vi "LVBlynk.vi"() -> ()   [LabVIEW 2014]
uses:
  utilities/BlynkLogs.vi
panel:
  in  "LED":bool
  out "Array":string[](array[string])
  in  "Notify":bool
  out "Log":string
  in  "Stop Button":bool
  out "Connected":bool
  in  "Auth Token from Blynk app":string="c3404b1e978b40fcbb409a59fc5da34b"
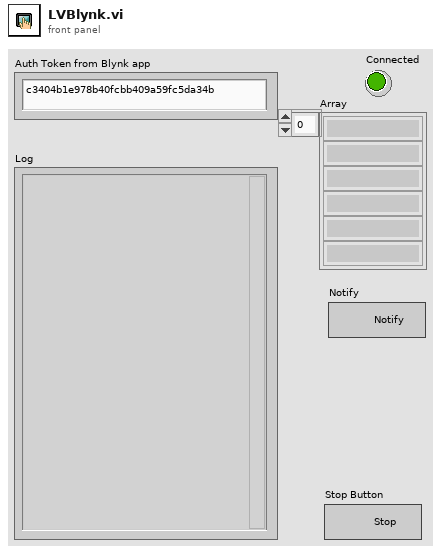
[diagram p1: front panel]
types:
  T1 = typedef "MsgType.ctl" = enum8{"RSP", "REGISTER", "LOGIN", "SAVE_PROF", "LOAD_PROF", "GET_TOKEN", "PING", "ACTIVATE", "DEACTIVATE", "REFRESH", "UNDEFINED0", "UNDEFINED1", "TWEET", "EMAIL", "NOTIFY", "BRIDGE", "UNDEFINED2", "UNDEFINED3", "UNDEFINED4", "UNDEFINED5", "HW"}
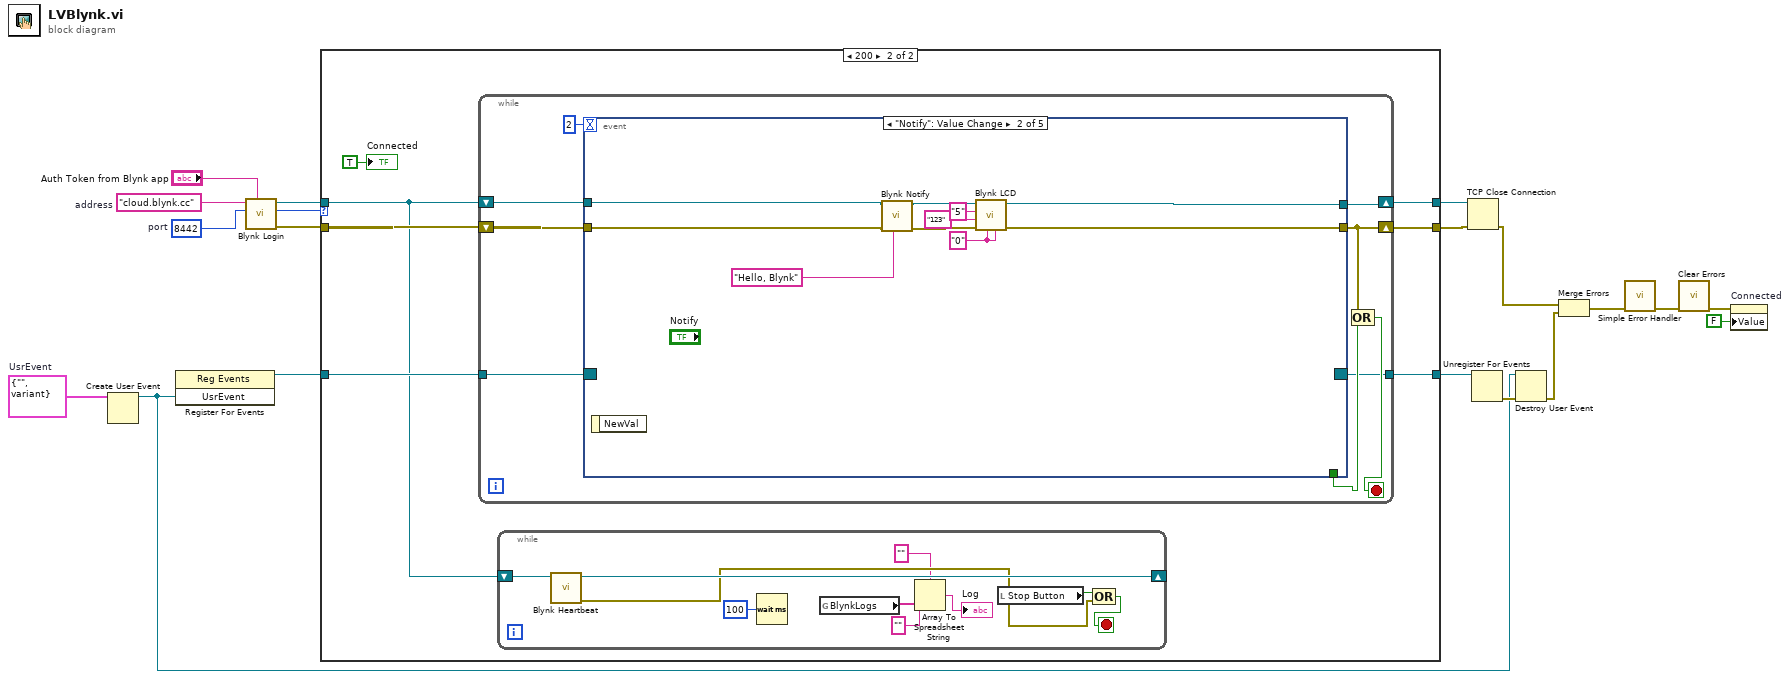
[diagram p0: block diagram]
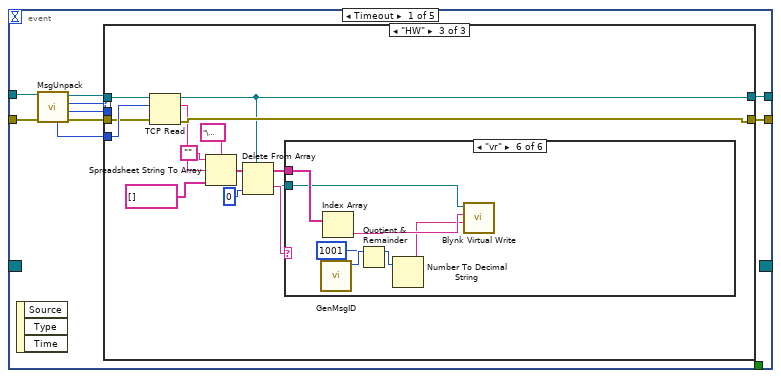
[diagram p3: hidden frame]
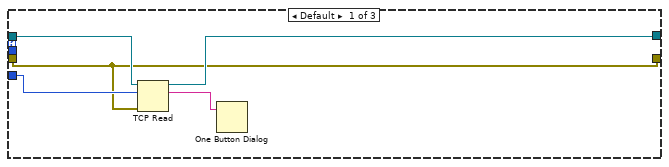
[diagram p4: hidden frame]
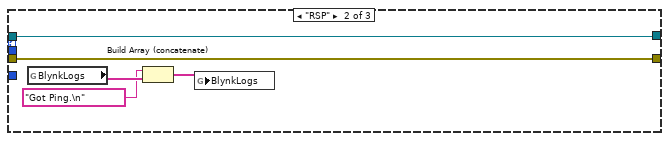
[diagram p5: hidden frame]
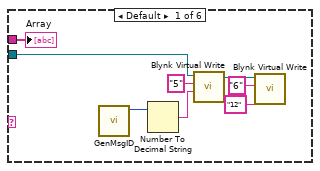
[diagram p6: hidden frame]
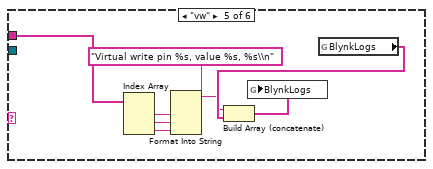
[diagram p10: hidden frame]
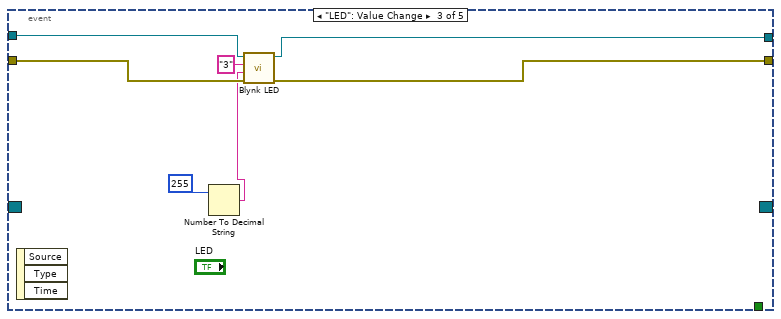
[diagram p11: hidden frame]
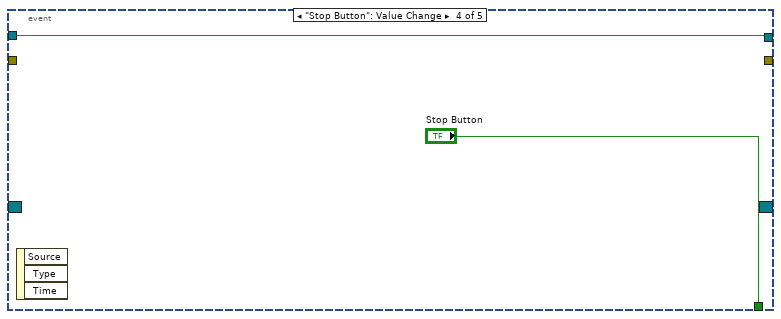
[diagram p12: hidden frame]
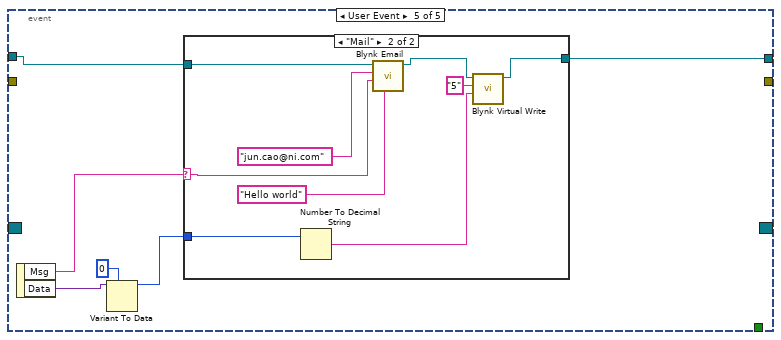
[diagram p13: hidden frame]
diagram:
  w5 = cluster{"Msg":string, "Data":variant} {"Msg"="", "Data"=variant}  # UsrEvent
  w15 = "cloud.blynk.cc"  # address
  w14 = u16 8442  # port
  n1 = Create User Event(user event datatype=w5) -> (user event=w4:refnum<user-event>)  [unwired: 1 in, 1 out]
  n2 = register-events(w4) -> (reference out=w8:refnum<event-registration>)  [unwired: 2 in, 1 out]
  n3 = call "Blynk Login.vi"("Auth Token"="Auth Token from Blynk app", "port (8442)"=w14, "address (cloud.blynk.cc)"=w15) -> ("error out"=w10:errorcluster, "STATUS"=w11:u16, "connection out"=w12:refnum<k5>)  [unwired: 6 in]
  n4 = case shown="200" w11 {
    tunnel: [w21 w28] -> w19
    tunnel: w12 -> [w21 w22]
    tunnel: [w20 w27] -> w18
    tunnel: w10 -> [w20 w24]
    tunnel: w8 -> [_ w26]
    tunnel: [_ w25] -> w7
    frame Default {
    }
    frame 200 {
      n5 = while {
        shift-right: [w46] -> w28
        shift-left: w22 -> [w39]
        shift-right: [w44] -> w27
        shift-left: w24 -> [w47]
        tunnel: w26 -> [w41]
        tunnel: [w40] -> w25
        stop <- w42 stop-if-true
        n6 = event shown="[1] \"Notify\": Value Change" {
          selector: w41 -> [_ _ _ _ _]
          dyn-events: [_ _ _ _ _] -> w40
          timeout: 2 -> [_ _ _ _ _]
          tunnel: w39 -> [w56 w112 w119 w120 w127]
          tunnel: w47 -> [w55 w111 w117 _ _]
          tunnel: [w51 w108 w118 w120 w126] -> w46
          tunnel: [w50 w103 w116 _ _] -> w44
          tunnel: [_ _ _ "Stop Button" _] -> w43
          event Timeout {
            n7 = event-data() -> ()  [unwired: 1 in, 3 out]
            n8 = call "MsgUnpack.vi"("error in (no error)"=w55, "connection"=w56) -> ("error out"=w52:errorcluster, "msg_id"=w48:u16, "msg_type"=w54:T1, "connection out"=w49:refnum<k5>, "msg_len"=w53:u16)  [unwired: 5 in]
            n9 = case shown="\"HW\"" w54 {
              tunnel: w49 -> [w59 w65 w79]
              tunnel: w53 -> [w61 _ w78]
              tunnel: w52 -> [w57 w66 w77]
              tunnel: [w57 w66 w76] -> w50
              tunnel: [w58 w65 w67] -> w51
              tunnel: w48 -> [_ _ _]
              frame Default {
                n10 = TCP Read(connection ID=w59, bytes to read=w61, error in (no error)=w57) -> (connection ID out=w58:refnum<k5>, data out=w60:string)  [unwired: 2 in, 1 out]
                n11 = One Button Dialog(message=w60) -> ()  [unwired: 1 in, 1 out]
              }
              frame "RSP" {
                n12 = global read "BlynkLogs.vi" "BlynkLogs"() -> (w64:string[])
                n13 = Build Array (concatenate)("Got Ping.\n" ("BlynkLogs"), w64) -> (w63:string[])
                n14 = global write "BlynkLogs.vi" "BlynkLogs"(w63) -> ()
              }
              frame "HW" {
                n15 = TCP Read(connection ID=w79, bytes to read=w78, error in (no error)=w77) -> (connection ID out=w67:refnum<k5>, data out=w75:string, error out=w76:errorcluster)  [unwired: 2 in]
                n16 = Spreadsheet String To Array(delimiter (Tab)="\u0000", format string="", spreadsheet string=w75, array type (2D Dbl)=string[] []) -> (array=w71:string[])
                n17 = Delete From Array(array=w71, index=0) -> (deleted portion=w70:string, array with subset deleted=w68:string[])  [unwired: 1 in]
                n18 = case shown="\"vr\"" w70 {
                  tunnel: w68 -> [w87 _ _ _ w95 w102]
                  tunnel: w67 -> [w86 _ _ _ _ w99]
                  frame Default {
                    n19 = call "GenMsgID.vi"() -> ("MsgID"=w81:u16)  [unwired: 10 in, 1 out]
                    n20 = Number To Decimal String(number=w81) -> (decimal integer string=w80:string)  [unwired: 1 in]
                    n21 = call "Blynk Virtual Write.vi"("value"=w80, "pin"="5", "connection"=w86) -> ("connection out"=w84:refnum<k5>)  [unwired: 7 in, 1 out]
                    n22 = call "Blynk Virtual Write.vi"("value"="12", "pin"="6", "connection"=w84) -> ()  [unwired: 7 in, 2 out]
                    "Array" <- w87
                  }
                  frame "info" {
                  }
                  frame "dw" {
                  }
                  frame "aw" {
                  }
                  frame "vw" {
                    n23 = Index Array(array=w95) -> (element #1=w94:string, element #2=w93:string, element #3=w91:string)  [unwired: 3 in]
                    n24 = Format Into String(format string="Virtual write pin %s, value %s, %s\\n", w94, w93, w91) -> (resulting string=w88:string)  [unwired: 2 in, 1 out]
                    n25 = global read "BlynkLogs.vi" "BlynkLogs"() -> (w90:string[])
                    n26 = Build Array (concatenate)(w88, w90) -> (w89:string[])
                    n27 = global write "BlynkLogs.vi" "BlynkLogs"(w89) -> ()
                  }
                  frame "vr" {
                    n28 = call "GenMsgID.vi"() -> ("MsgID"=w98:u16)  [unwired: 10 in, 1 out]
                    n29 = Index Array(array=w102) -> (element=w101:string)  [unwired: 1 in]
                    n30 = Quotient & Remainder(x=w98, y=u16 1001) -> (x-y*floor(x/y)=w96:u16)  [unwired: 1 out]
                    n31 = Number To Decimal String(number=w96) -> (decimal integer string=w100:string)  [unwired: 1 in]
                    n32 = call "Blynk Virtual Write.vi"("value"=w100, "pin"=w101, "connection"=w99) -> ()  [unwired: 7 in, 2 out]
                  }
                }
              }
            }
          }
          event "Notify": Value Change {
            w105 = "0" ("coord_x")
            n33 = event-data() -> ()  [unwired: 1 in, 1 out]
            n34 = call "Blynk Notify.vi"("message"="Hello, Blynk", "error in (no error)"=w111, "connection"=w112) -> ("error out"=w107:errorcluster, "connection out"=w109:refnum<k5>)  [unwired: 7 in]
            n35 = call "Blynk LCD.vi"("coord_y"=w105, "coord_x"=w105, "error in"=w107, "value"="123", "pin"="5", "connection"=w109) -> ("error out"=w103:errorcluster, "connection out"=w108:refnum<k5>)  [unwired: 4 in]
          }
          event "LED": Value Change {
            n36 = event-data() -> ()  [unwired: 1 in, 3 out]
            n37 = Number To Decimal String(number=u8 255) -> (decimal integer string=w113:string)  [unwired: 1 in]
            n38 = call "Blynk LED.vi"("error in (no error)"=w117, "value"=w113, "pin"="3", "connection"=w119) -> ("error out"=w116:errorcluster, "connection out"=w118:refnum<k5>)  [unwired: 6 in]
          }
          event "Stop Button": Value Change {
            n39 = event-data() -> ()  [unwired: 1 in, 3 out]
          }
          event User Event {
            n40 = event-data() -> ("Msg"=w125:string, "Data"=w124:variant)  [unwired: 1 in]
            n41 = Variant To Data(type=0, Variant=w124) -> (data=w122:i32)  [unwired: 1 in, 1 out]
            n42 = case shown="\"Mail\"" w125 {
              selector: w125 -> [_ w134]
              tunnel: w127 -> [w128 w135]
              tunnel: [w128 w132] -> w126
              tunnel: w122 -> [_ w130]
              frame "False", Default {
              }
              frame "Mail" {
                n43 = Number To Decimal String(number=w130) -> (decimal integer string=w129:string)  [unwired: 1 in]
                n44 = call "Blynk Email.vi"("message"="Hello world", "topic"=w134, "to"="jun.cao@ni.com", "connection"=w135) -> ("connection out"=w133:refnum<k5>)  [unwired: 6 in, 1 out]
                n45 = call "Blynk Virtual Write.vi"("value"=w129, "pin"="5", "connection"=w133) -> ("connection out"=w132:refnum<k5>)  [unwired: 7 in, 1 out]
              }
            }
          }
        }
        n46 = Compound Arithmetic op=OR(w44, w43) -> (w42:bool)
      }
      n47 = while {
        shift-right: [w37] -> _
        shift-left: w22 -> [w38]
        stop <- w30 stop-if-true
        n48 = call "Blynk Heartbeat.vi"("connection"=w38) -> ("error out"=w31:errorcluster, "connection out"=w37:refnum<k5>)  [unwired: 9 in]
        n49 = Wait (ms)(milliseconds to wait=u32 100) -> ()  [unwired: 1 out]
        n50 = global read "BlynkLogs.vi" "BlynkLogs"() -> (w34:string[])
        n51 = Array To Spreadsheet String(delimiter (Tab)="", array=w34, 3:"" ("format string")) -> (spreadsheet string=→"Log":string)
        n52 = local read "Stop Button"() -> (w32:bool)
        n53 = Compound Arithmetic op=OR(w32, w31) -> (w30:bool)
      }
      "Connected" <- TRUE ("Connected")
    }
  }
  n54 = TCP Close Connection(connection ID=w19, error in (no error)=w18) -> (error out=w3:errorcluster)  [unwired: 1 in, 1 out]
  n55 = Unregister For Events(event registration refnum=w7) -> (error out=w6:errorcluster)  [unwired: 1 in]
  n56 = Destroy User Event(user event=w4, error in=w6) -> (error out=w2:errorcluster)
  n57 = Merge Errors(w3, w2) -> (w1:errorcluster)
  n58 = call <vilib>:"Simple Error Handler.vi"("error in (no error)"=w1) -> ("error out"=w17:errorcluster)  [unwired: 4 in, 4 out]
  n59 = call <vilib>:"Clear Errors.vi"("error in (no error)"=w17) -> ("error out"=w9:errorcluster)  [unwired: 5 in, 1 out]
  n60 = property on="Connected" class="Bool (strict)"(error in=w9, "Value"=FALSE ("Connected")) -> ()  [unwired: 1 in, 2 out]
